vi "1_ACTIVEX_covid_19.vi"() -> ()   [LabVIEW 2019]
panel:
  in  "WindowsMediaPlayer":refnum<k7>(container)
  in  "WebBrowser":refnum<k7>(container)
  in  "String":string
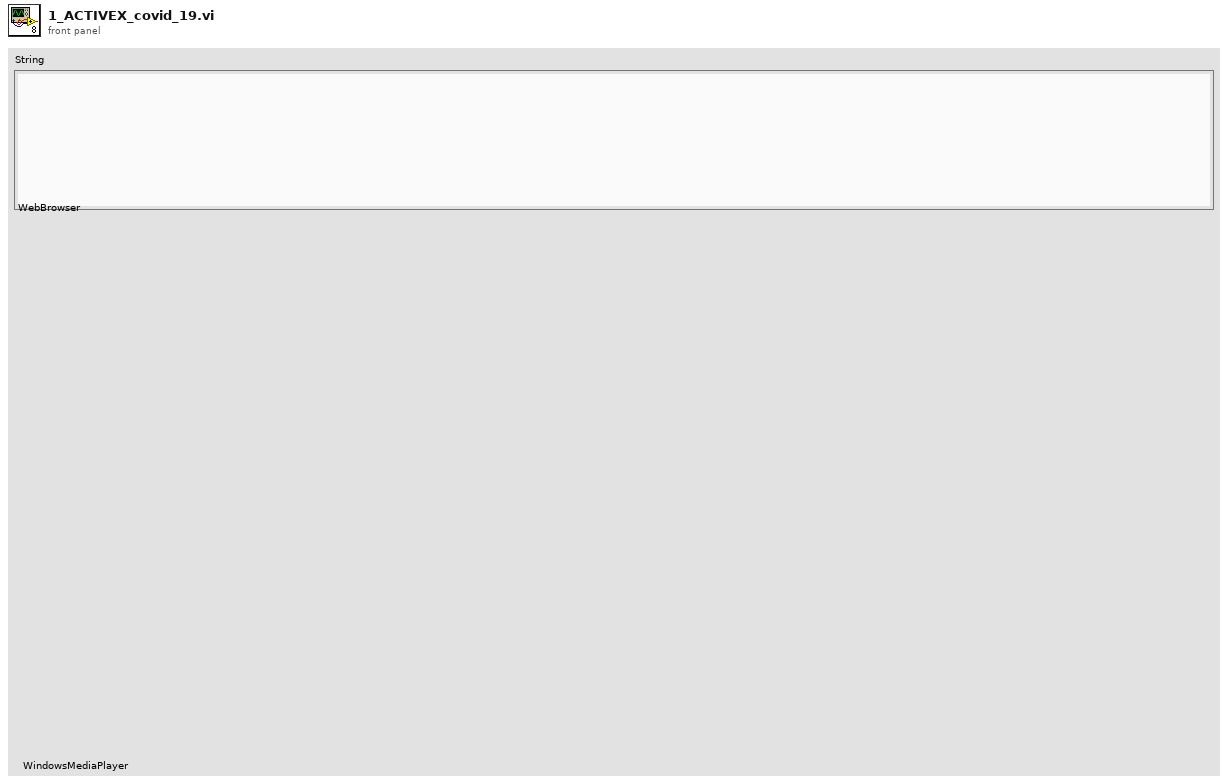
[diagram p1: front panel]
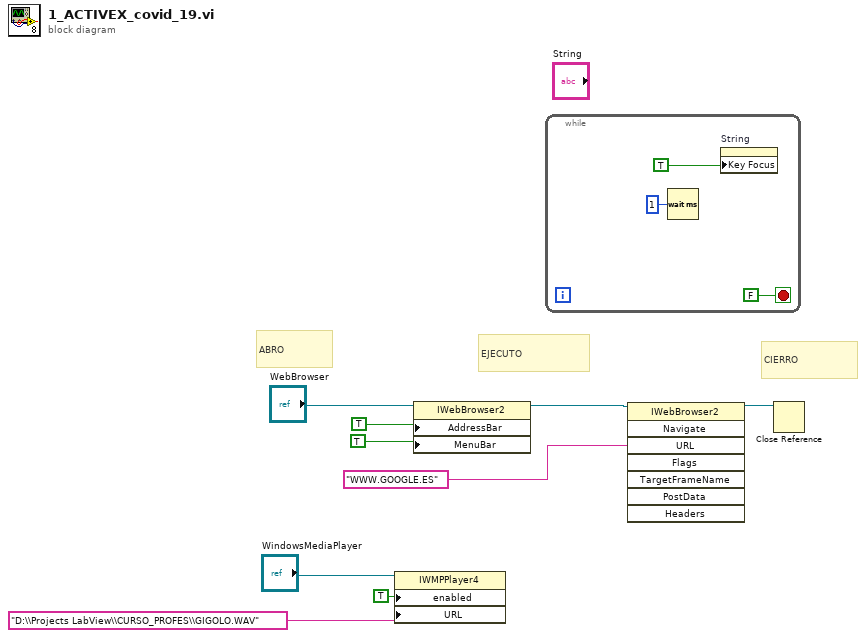
[diagram p0: block diagram]
diagram:
  # "EJECUTO"
  # "CIERRO"
  # "ABRO"
  n1 = property class="IWMPPlayer4"(reference="WindowsMediaPlayer", "enabled"=TRUE, "URL"="D:\\Projects LabView\\CURSO_PROFES\\GIGOLO.WAV") -> ()  [unwired: 1 in, 2 out]
  n2 = property class="IWebBrowser2"(reference="WebBrowser", "AddressBar"=TRUE, "MenuBar"=TRUE ("AddressBar")) -> (reference out=w6:refnum<k7>)  [unwired: 1 in, 1 out]
  n3 = while {
    stop <- FALSE stop-if-true
    n4 = Wait (ms)(milliseconds to wait=u32 1) -> ()  [unwired: 1 out]
    n5 = property on="String" class="Str"("Key Focus"=TRUE) -> ()  [unwired: 2 in, 2 out]
  }
  n6 = invoke class="IWebBrowser2" method="Navigate"(reference=w6, "URL"="WWW.GOOGLE.ES") -> (reference out=w4:refnum<k7>)  [unwired: 6 in, 7 out]
  n7 = Close Reference(reference=w4) -> ()  [unwired: 1 in, 1 out]
